vi "make_scene_main.vi"(1 "All Properties":T9, 5 "Scene Objects In":T2, 7 "Graph Properties":T1, 9 "Plot Processed Data":T3={"Plot Rep Arrays"=[], "Graph Range Min/Max"={"X"={"Min"=0.0, "Max"=-inf}, "Y"={"Min"=0.0, "Max"=-inf}, "Z"={"Min"=inf, "Max"=-inf}, "Amplitude"={"Min"=0.0, "Max"=0.0}}}, 12 "Update?":T35, 14 "Track Eye":T34) -> (6 "Scene Objects Out":T2, 10 "Translate By":T33, 15 "Scale By":T33)   [LabVIEW 2020, in "3DPC_SurfacePlot.xctl"]
uses:
  <vilib>/Native 3D Graph/xcontrol/3DPC_SurfacePlot.xctl
  <vilib>/Native 3D Graph/typedefs/vector.ctl
  <vilib>/Native 3D Graph/typedefs/update_scene_all.ctl
  <vilib>/Native 3D Graph/typedefs/update_scene_component.ctl
  <vilib>/Native 3D Graph/typedefs/track_eye.ctl
  <vilib>/Native 3D Graph/typedefs/all_non_graph_prop.ctl
  <vilib>/Native 3D Graph/typedefs/prop_plot_all_array.ctl
  <vilib>/Native 3D Graph/typedefs/prop_plot_all.ctl
  <vilib>/Native 3D Graph/typedefs/prop_plot_projection.ctl
  <vilib>/Native 3D Graph/typedefs/prop_plot_surface.ctl
  <vilib>/Native 3D Graph/typedefs/prop_plot_contour.ctl
  <vilib>/Native 3D Graph/typedefs/prop_plot_normal.ctl
  <vilib>/Native 3D Graph/typedefs/prop_plot_point_line.ctl
  <vilib>/Native 3D Graph/typedefs/prop_value_pair_all.ctl
  <vilib>/Native 3D Graph/typedefs/prop_value_pair_1d.ctl
  <vilib>/Native 3D Graph/typedefs/prop_axes_all.ctl
  <vilib>/Native 3D Graph/typedefs/prop_axes_grid.ctl
  <vilib>/Native 3D Graph/typedefs/prop_axes_ticks.ctl
  <vilib>/Native 3D Graph/typedefs/range_cluster.ctl
  <vilib>/Native 3D Graph/typedefs/min_max.ctl
  <vilib>/Native 3D Graph/typedefs/prop_axes_captions.ctl
  <vilib>/Native 3D Graph/typedefs/prop_axes_labels.ctl
  <vilib>/Native 3D Graph/typedefs/prop_axes_autorange.ctl
  <vilib>/Native 3D Graph/typedefs/prop_cursor_all_array.ctl
  <vilib>/Native 3D Graph/typedefs/prop_cursor_point.ctl
  <vilib>/Native 3D Graph/typedefs/prop_cursor_position.ctl
  <vilib>/Native 3D Graph/typedefs/prop_cursor_line.ctl
  <vilib>/Native 3D Graph/typedefs/prop_cursor_plane.ctl
  <vilib>/Native 3D Graph/typedefs/prop_cursor_text.ctl
  <vilib>/Native 3D Graph/typedefs/prop_format.ctl
  <vilib>/Native 3D Graph/typedefs/prop_lighting.ctl
  <vilib>/Native 3D Graph/typedefs/plot_processed_data.ctl
  <vilib>/Native 3D Graph/typedefs/plot_rep_array.ctl
  <vilib>/Native 3D Graph/typedefs/plot_rep.ctl
  <vilib>/Native 3D Graph/typedefs/plot_rep_mesh_data.ctl
  <vilib>/Native 3D Graph/typedefs/state_scene_objects.ctl
  <vilib>/Native 3D Graph/typedefs/prop_graph.ctl
  <vilib>/picture/3D Picture Control/Object/Create Object (name).vi
  <vilib>/picture/3D Picture Control/NI_3D Picture Control.lvlib
panel:
  out "Scene Objects Out":T2
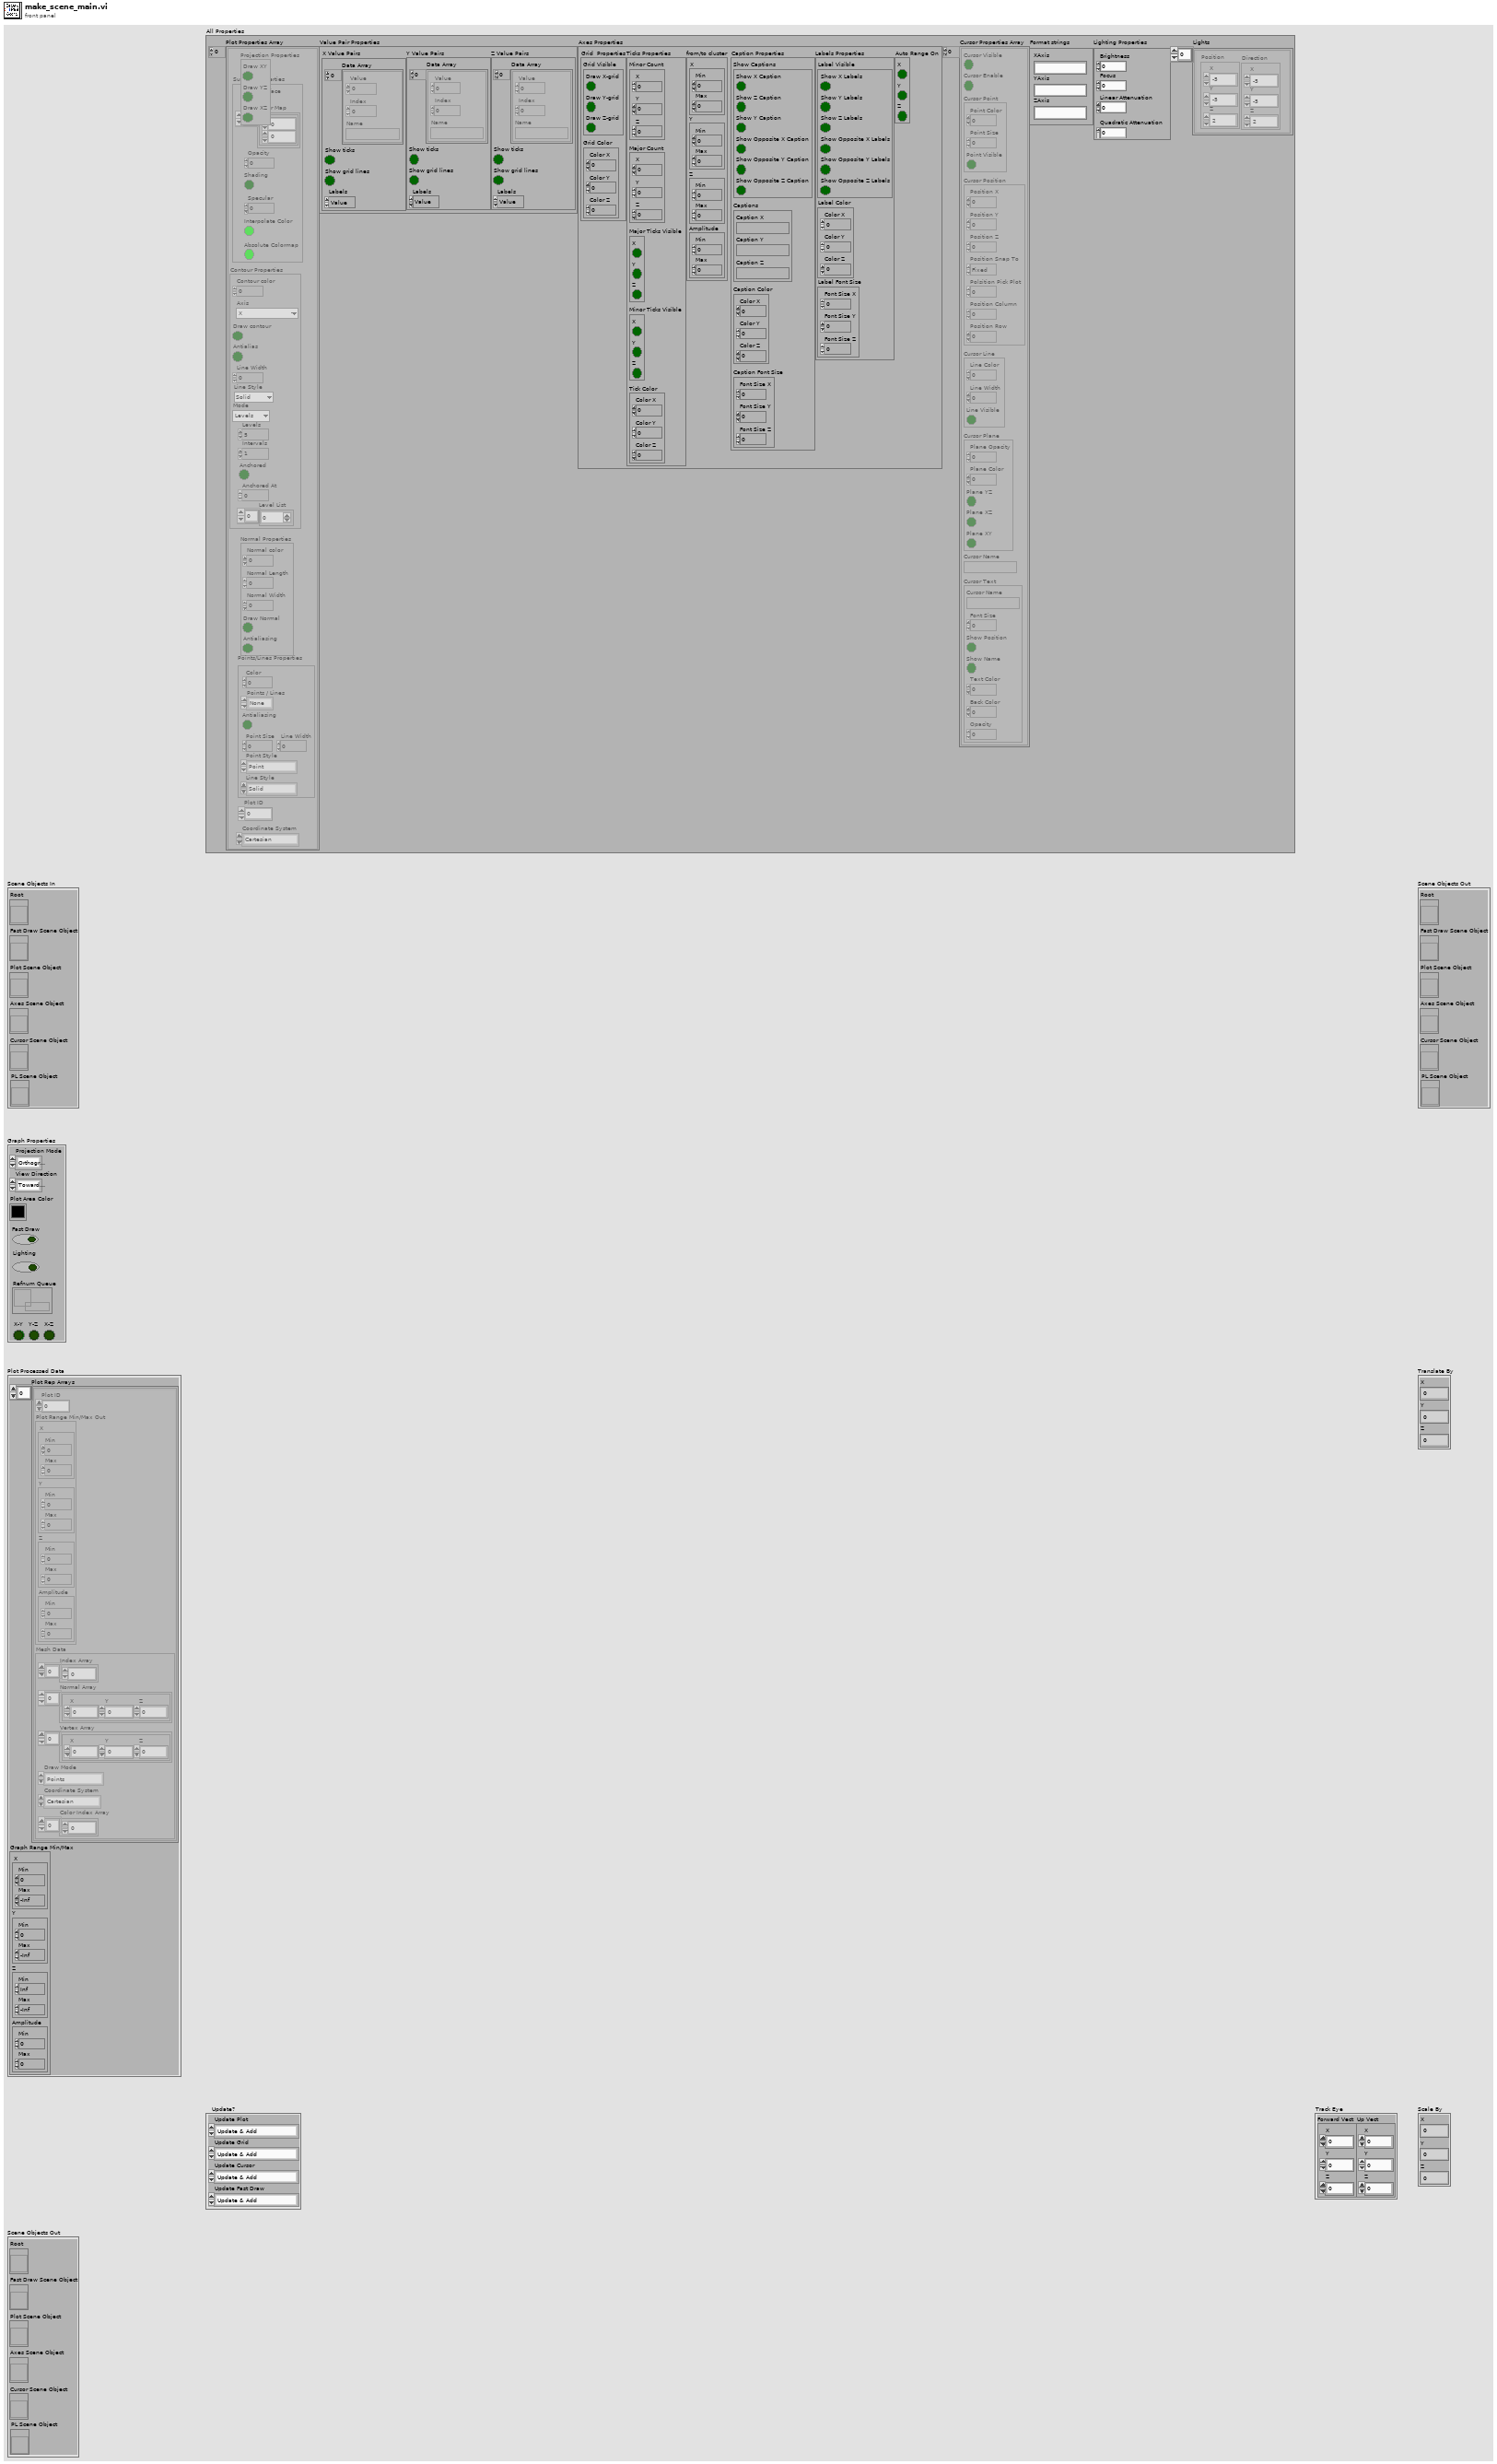
[diagram p1: front panel]
types:
  T1 = typedef "3DPC_SurfacePlot.xctl/prop_graph.ctl" = cluster{"Projection Mode":enum16{"Orthographic", "Perspective"}, "View Direction":enum32{"Towards X-Y Plane", "Towards Y-Z Plane", "Towards X-Z Plane", "User Define"}, "Plot Area Color":u32, "Fast Draw":bool, "X-Y":bool, "Y-Z":bool, "X-Z":bool, "Lighting":bool, "Refnum Queue":refnum<queue>}
  T2 = typedef "3DPC_SurfacePlot.xctl/state_scene_objects.ctl" = cluster{"Root":refnum<vi>, "Fast Draw Scene Object":refnum<vi>, "Plot Scene Object":refnum<vi>, "Axes Scene Object":refnum<vi>, "Cursor Scene Object":refnum<vi>, "PL Scene Object":refnum<vi>}
  T3 = typedef "plot_processed_data.ctl" = cluster{"Plot Rep Arrays":T4, "Graph Range Min/Max":T6}
  T4 = typedef "3DPC_SurfacePlot.xctl/plot_rep_array.ctl" = T5[]
  T5 = typedef "3DPC_SurfacePlot.xctl/plot_rep.ctl" = cluster{"Plot ID":i32, "Plot Range Min/Max Out":T6, "Mesh Data":T8}
  T6 = typedef "3DPC_SurfacePlot.xctl/range_cluster.ctl" = cluster{"X":T7, "Y":T7, "Z":T7, "Amplitude":T7}
  T7 = typedef "3DPC_SurfacePlot.xctl/min_max.ctl" = cluster{"Min":sgl, "Max":sgl}
  T8 = typedef "3DPC_SurfacePlot.xctl/plot_rep_mesh_data.ctl" = cluster{"Index Array":u32[], "Normal Array":cluster{"X":sgl, "Y":sgl, "Z":sgl}[], "Vertex Array":cluster{"X":sgl, "Y":sgl, "Z":sgl}[], "Draw Mode":enum16{"Points", "Lines", "Line Strip", "Line Loop", "Triangles", "Triangle Strip", "Triangle Fan", "Quads", "Quad Strip", "Polygon"}, "Coordinate System":enum16{"Cartesian", "Cylindrical", "Spherical"}, "Color Index Array":i32[]}
  T9 = typedef "3DPC_SurfacePlot.xctl/all_non_graph_prop.ctl" = cluster{"Plot Properties Array":T10, "Value Pair Properties":T17, "Axes Properties":T19, "Cursor Properties Array":T25, "Format strings":T31, "Lighting Properties":T32, "Lights":cluster{"Position":cluster{"X":sgl, "Y":sgl, "Z":sgl}, "Direction":cluster{"X":sgl, "Y":sgl, "Z":sgl}}[]}
  T10 = typedef "3DPC_SurfacePlot.xctl/prop_plot_all_array.ctl" = T11[]
  T11 = typedef "3DPC_SurfacePlot.xctl/prop_plot_all.ctl" = cluster{"Projection Properties":T12, "Surface Properties":T13, "Contour Properties":T14, "Normal Properties":T15, "Points/Lines Properties":T16, "Plot ID":i32, "Coordinate System":enum16{"Cartesian", "Cylindrical", "Spherical"}}
  T12 = typedef "3DPC_SurfacePlot.xctl/prop_plot_projection.ctl" = cluster{"Draw XY":bool, "Draw YZ":bool, "Draw XZ":bool}
  T13 = typedef "3DPC_SurfacePlot.xctl/prop_plot_surface.ctl" = cluster{"Draw surface":bool, "Opacity":dbl, "Shading":bool, "Specular":i32, "Color Map":cluster{dbl, u32}[], "Interpolate Color":bool, "Absolute Colormap":bool}
  T14 = typedef "3DPC_SurfacePlot.xctl/prop_plot_contour.ctl" = cluster{"Contour color":u32, "Axis":enum16{"X", "Y", "Z"}, "Draw contour":bool, "Antialias":bool, "Line Width":sgl, "Contour Line Style":enum16{"Solid", "Dash", "Dot", "Dash Dot"}, "Mode":enum16{"Levels", "Intervals", "Level List"}, "Levels":sgl, "Intervals":sgl, "Anchored At":sgl, "Anchored":bool, "Level List":dbl[]}
  T15 = typedef "3DPC_SurfacePlot.xctl/prop_plot_normal.ctl" = cluster{"Normal color":u32, "Normal Length":sgl, "Normal Width":sgl, "Draw Normal":bool, "Antialiasing":bool}
  T16 = typedef "3DPC_SurfacePlot.xctl/prop_plot_point_line.ctl" = cluster{"Color":u32, "Antialiasing":bool, "Point Size":sgl, "Points / Lines":enum16{"None", "Points", "Lines", "Both"}, "Point Style":enum16{"Point", "EmptySquare", "Asterisk", "Diamond", "EmptyCircle", "Circle", "X"}, "Line Style":enum16{"Solid", "Dash", "Dot", "Dash Dot"}, "Line Width":sgl}
  T17 = typedef "3DPC_SurfacePlot.xctl/prop_value_pair_all.ctl" = cluster{"X Value Pairs":cluster{"Data Array":cluster{"Value":sgl, "Index":i32, "Name":string}[], "Show ticks":bool, "Show grid lines":bool, "Labels":enum16{"Value", "None", "Name"}}, "Y Value Pairs":T18, "Z Value Pairs":T18}
  T18 = typedef "3DPC_SurfacePlot.xctl/prop_value_pair_1d.ctl" = cluster{"Data Array":cluster{"Value":sgl, "Index":i32, "Name":string}[], "Show ticks":bool, "Show grid lines":bool, "Labels":enum16{"Value", "None", "Name"}}
  T19 = typedef "3DPC_SurfacePlot.xctl/prop_axes_all.ctl" = cluster{"Grid  Properties":T20, "Ticks Properties":T21, "from/to cluster":T6, "Caption Properties":T22, "Labels Properties":T23, "Auto Range On":T24}
  T20 = typedef "3DPC_SurfacePlot.xctl/prop_axes_grid.ctl" = cluster{"Grid Visible":cluster{"Draw X-grid":bool, "Draw Y-grid":bool, "Draw Z-grid":bool}, "Grid Color":cluster{"Color X":u32, "Color Y":u32, "Color Z":u32}}
  T21 = typedef "3DPC_SurfacePlot.xctl/prop_axes_ticks.ctl" = cluster{"Minor Count":cluster{"X":i32, "Y":i32, "Z":i32}, "Major Count":cluster{"X":i32, "Y":i32, "Z":i32}, "Major Ticks Visible":cluster{"X":bool, "Y":bool, "Z":bool}, "Minor Ticks Visible":cluster{"X":bool, "Y":bool, "Z":bool}, "Tick Color":cluster{"Color X":u32, "Color Y":u32, "Color Z":u32}}
  T22 = typedef "3DPC_SurfacePlot.xctl/prop_axes_captions.ctl" = cluster{"Show Captions":cluster{"Show X Caption":bool, "Show Z Caption":bool, "Show Y Caption":bool, "Show Opposite X Caption":bool, "Show Opposite Y Caption":bool, "Show Opposite Z Caption":bool}, "Captions":cluster{"Caption X":string, "Caption Y":string, "Caption Z":string}, "Caption Color":cluster{"Color X":u32, "Color Y":u32, "Color Z":u32}, "Caption Font Size":cluster{"Font Size X":i16, "Font Size Y":i16, "Font Size Z":i16}}
  T23 = typedef "3DPC_SurfacePlot.xctl/prop_axes_labels.ctl" = cluster{"Label Visible":cluster{"Show X Labels":bool, "Show Y Labels":bool, "Show Z Labels":bool, "Show Opposite X Labels":bool, "Show Opposite Y Labels":bool, "Show Opposite Z Labels":bool}, "Label Color":cluster{"Color X":u32, "Color Y":u32, "Color Z":u32}, "Label Font Size":cluster{"Font Size X":i16, "Font Size Y":i16, "Font Size Z":i16}}
  T24 = typedef "3DPC_SurfacePlot.xctl/prop_axes_autorange.ctl" = cluster{"X":bool, "Y":bool, "Z":bool}
  T25 = typedef "3DPC_SurfacePlot.xctl/prop_cursor_all_array.ctl" = cluster{"Cursor Visible":bool, "Cursor Enable":bool, "Cursor Point":T26, "Cursor Position":T27, "Cursor Line":T28, "Cursor Plane":T29, "Cursor Name":string, "Cursor Text":T30}[]
  T26 = typedef "3DPC_SurfacePlot.xctl/prop_cursor_point.ctl" = cluster{"Point Color":u32, "Point Size":dbl, "Point Visible":bool}
  T27 = typedef "3DPC_SurfacePlot.xctl/prop_cursor_position.ctl" = cluster{"Position X":dbl, "Position Y":dbl, "Position Z":dbl, "Position Snap To":enum16{"Fixed", "Nearest Plot", "Snap to Plot"}, "Polsition Pick Plot":u16, "Position Column":i32, "Position Row":i32}
  T28 = typedef "3DPC_SurfacePlot.xctl/prop_cursor_line.ctl" = cluster{"Line Color":u32, "Line Width":dbl, "Line Visible":bool}
  T29 = typedef "3DPC_SurfacePlot.xctl/prop_cursor_plane.ctl" = cluster{"Plane Opacity":dbl, "Plane Color":u32, "Plane YZ":bool, "Plane XZ":bool, "Plane XY":bool}
  T30 = typedef "3DPC_SurfacePlot.xctl/prop_cursor_text.ctl" = cluster{"Cursor Name":string, "Font Size":i32, "Show Position":bool, "Show Name":bool, "Text Color":u32, "Back Color":u32, "Opacity":dbl}
  T31 = typedef "3DPC_SurfacePlot.xctl/prop_format.ctl" = cluster{"XAxis":string, "YAxis":string, "ZAxis":string}
  T32 = typedef "3DPC_SurfacePlot.xctl/prop_lighting.ctl" = cluster{"Brightness":i32, "Focus":dbl, "Linear Attenuation":dbl, "Quadratic Attenuation":dbl}
  T33 = typedef "3DPC_SurfacePlot.xctl/vector.ctl" = cluster{"X":sgl, "Y":sgl, "Z":sgl}
  T34 = typedef "3DPC_SurfacePlot.xctl/track_eye.ctl" = cluster{"Forward Vect":T33, "Up Vect":T33}
  T35 = typedef "3DPC_SurfacePlot.xctl/update_scene_all.ctl" = cluster{"Update Plot":T36, "Update Grid":T36, "Update Cursor":T36, "Update Fast Draw":T36}
  T36 = typedef "3DPC_SurfacePlot.xctl/update_scene_component.ctl" = enum16{"Update & Add", "Update & Not Add", "Remove ", "Nothing", "Add"}
  T37 = cluster{"Position":cluster{"X":sgl, "Y":sgl, "Z":sgl}, "Direction":cluster{"X":sgl, "Y":sgl, "Z":sgl}}[]
  T38 = enum16{"Points", "Lines", "Line Strip", "Line Loop", "Triangles", "Triangle Strip", "Triangle Fan", "Quads", "Quad Strip", "Polygon"}
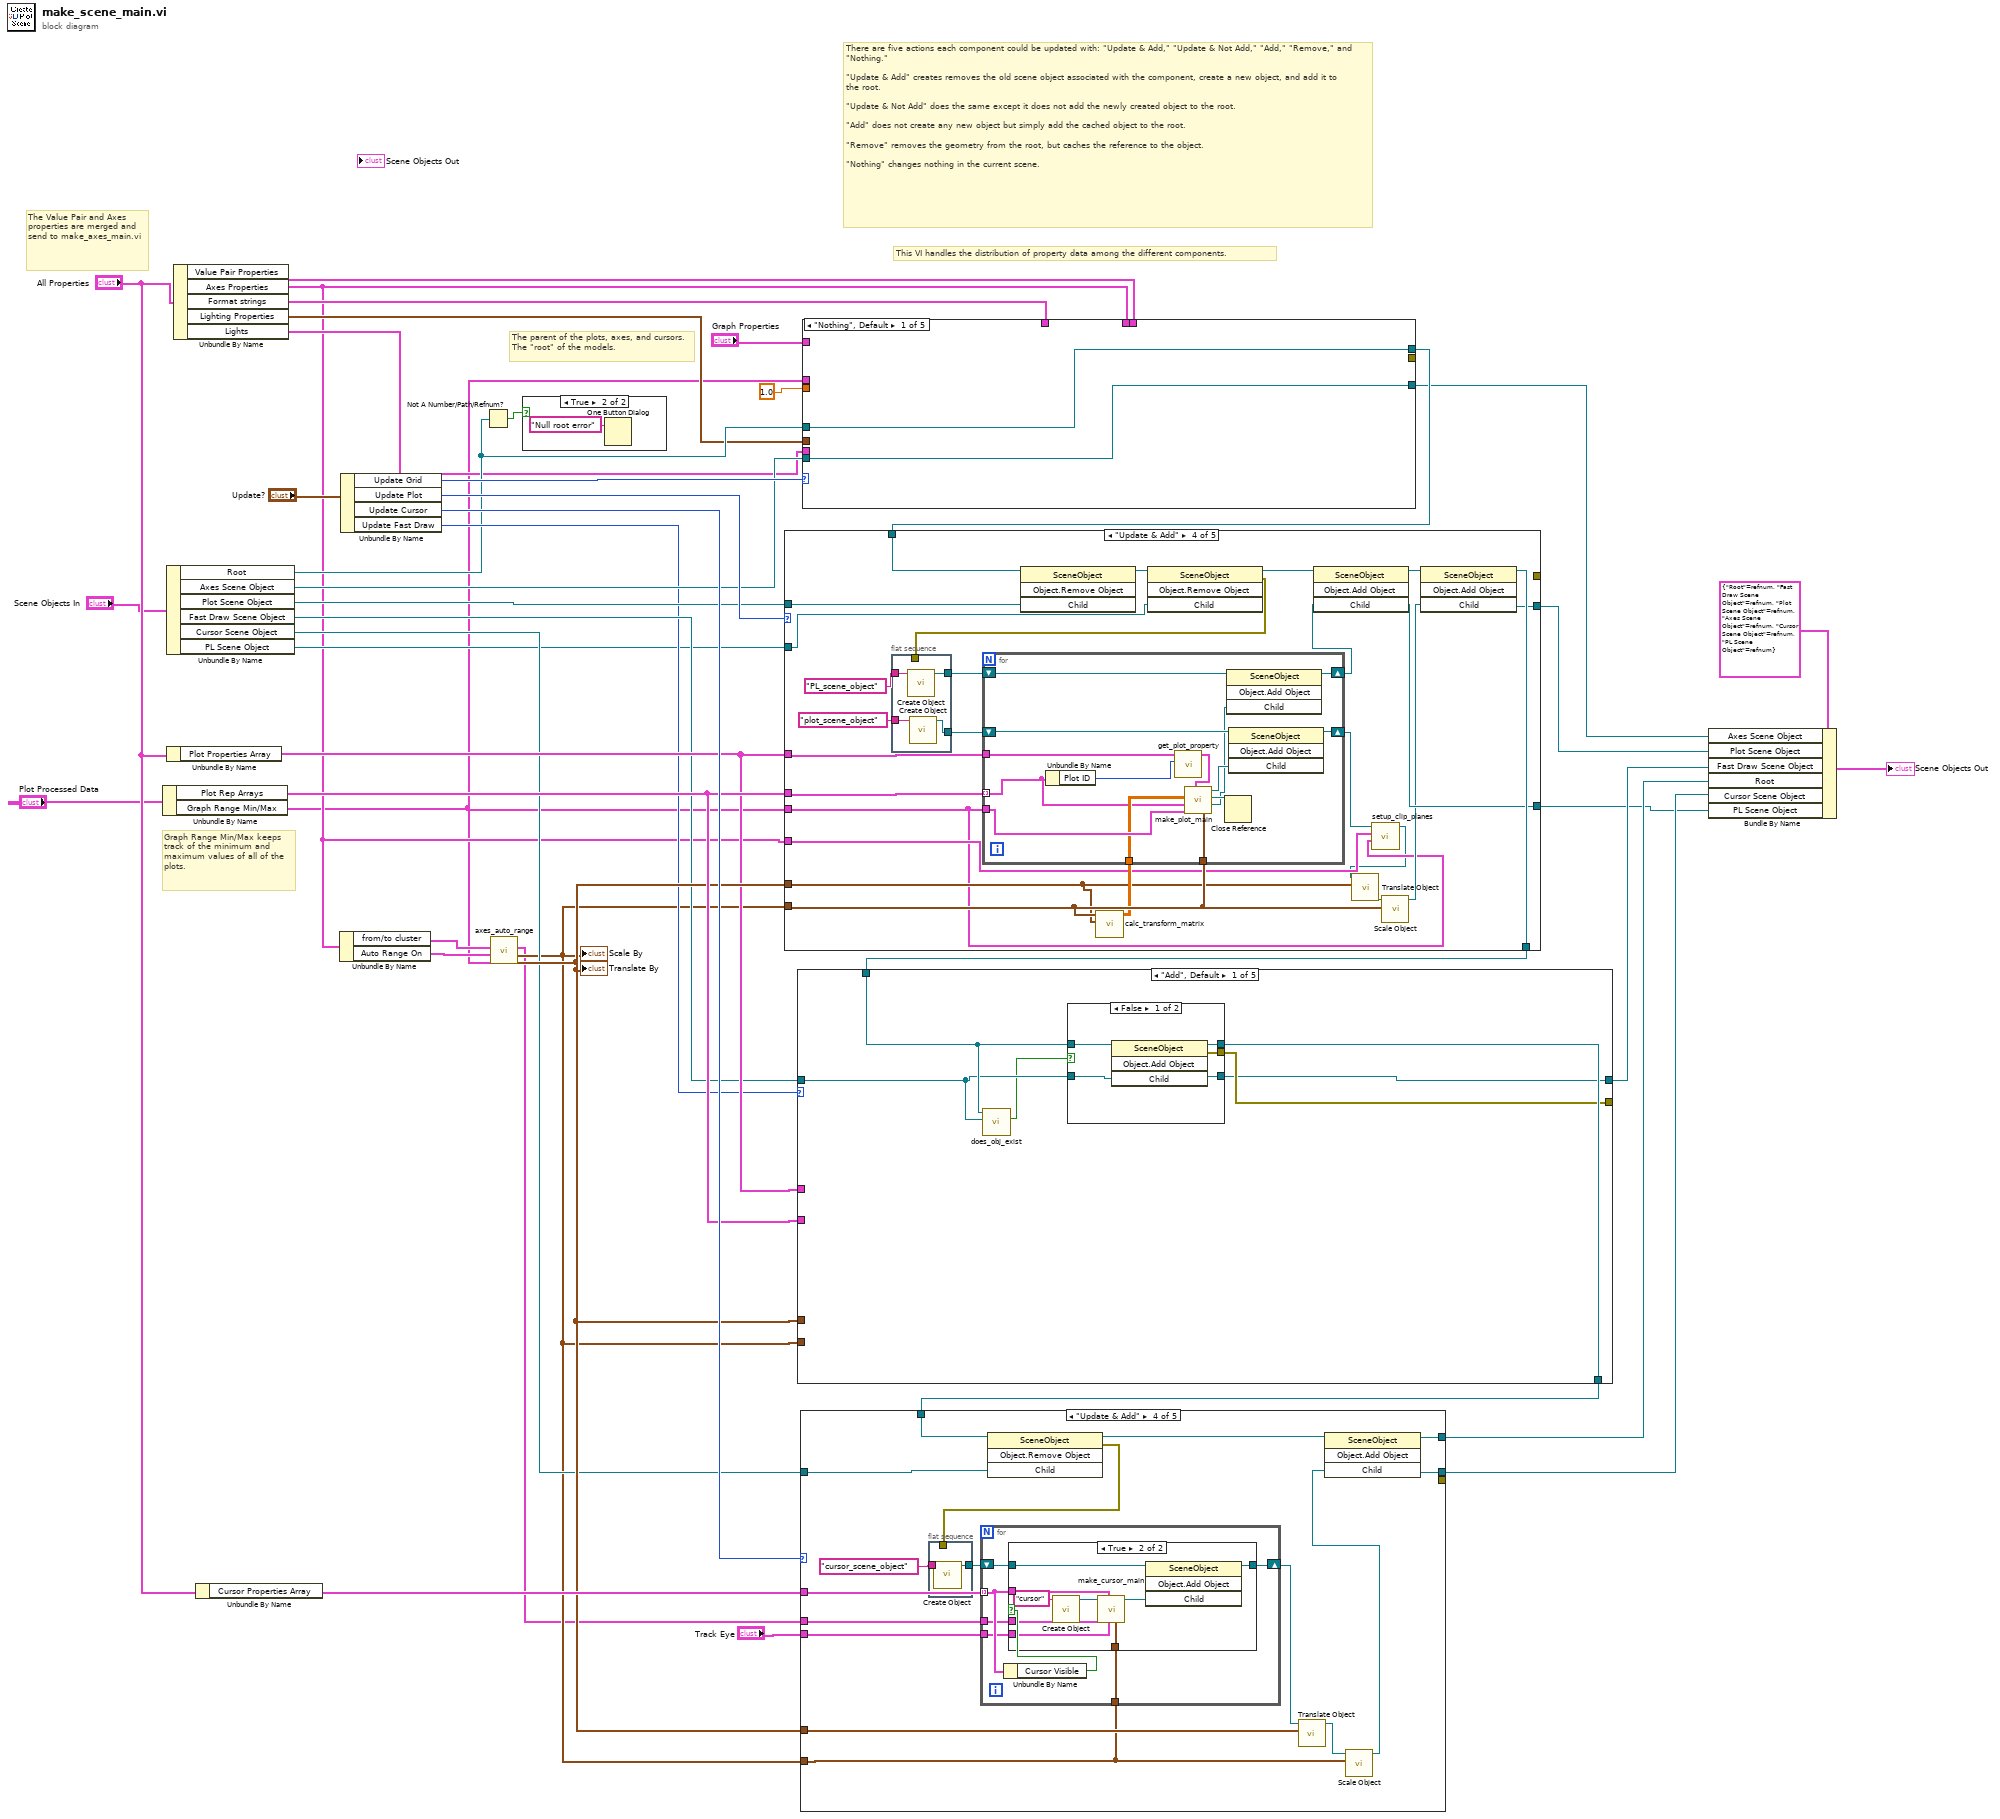
[diagram p0: block diagram]
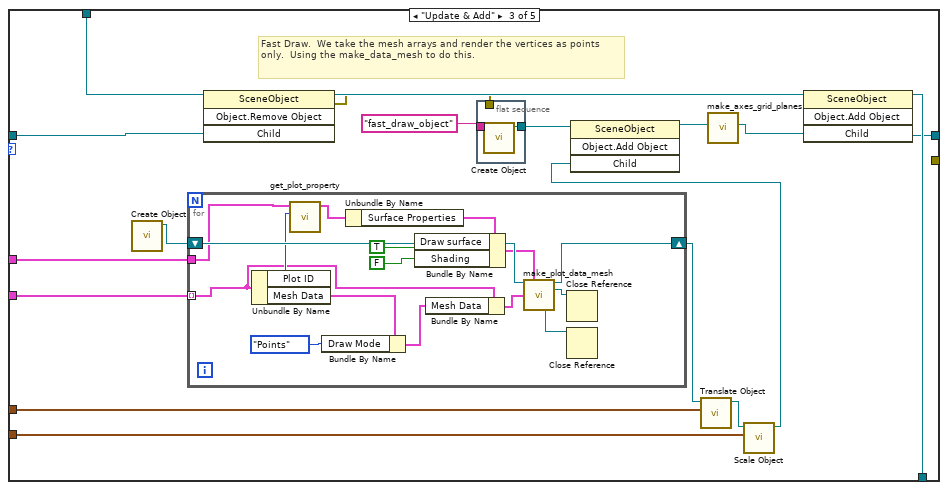
[diagram p5: hidden frame]
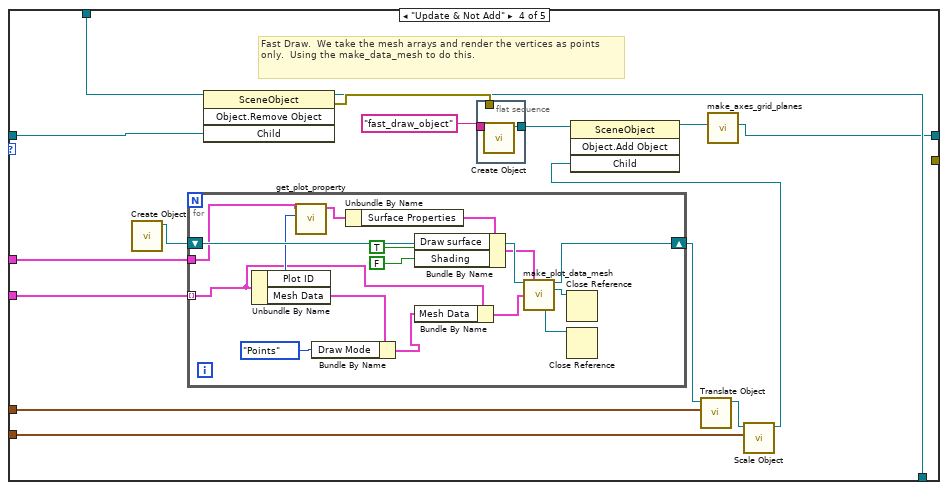
[diagram p6: hidden frame]
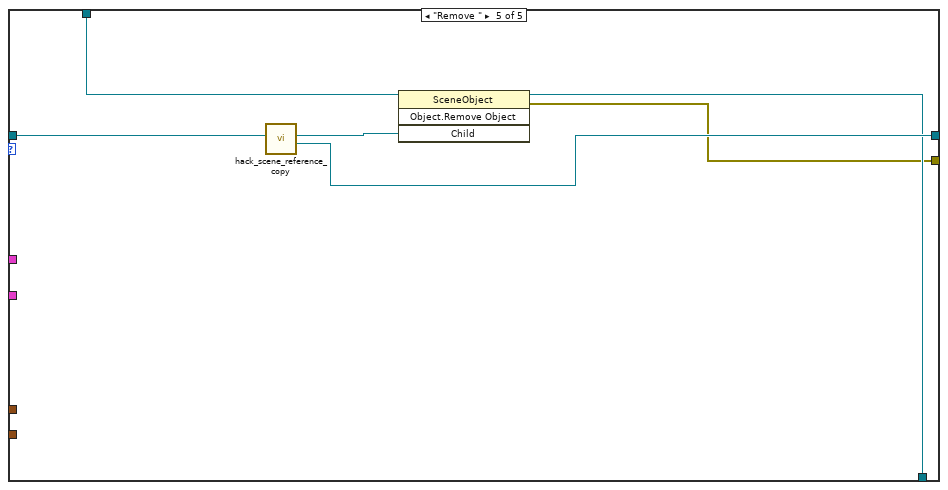
[diagram p7: hidden frame]
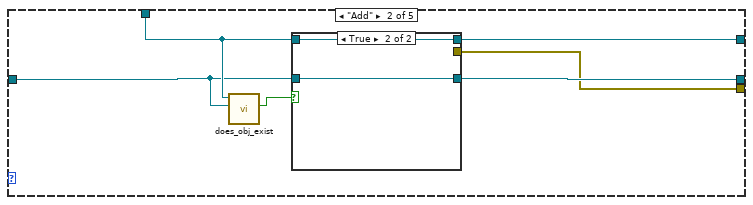
[diagram p9: hidden frame]
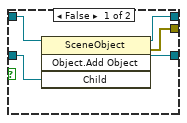
[diagram p10: hidden frame]
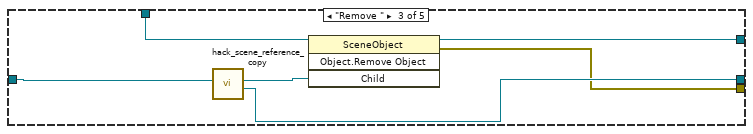
[diagram p11: hidden frame]
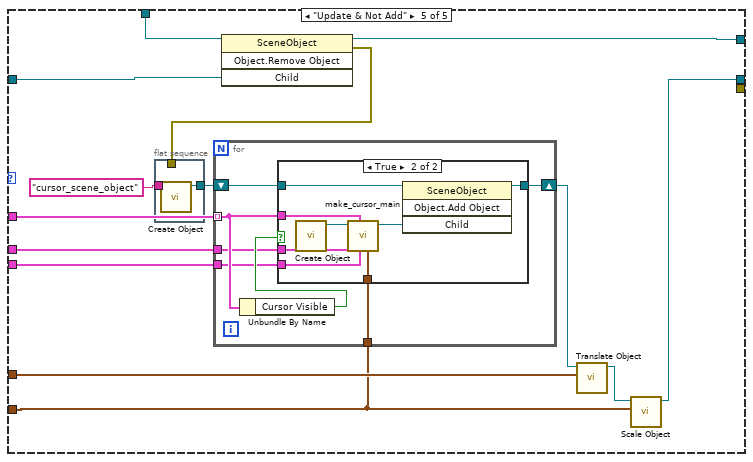
[diagram p13: hidden frame]
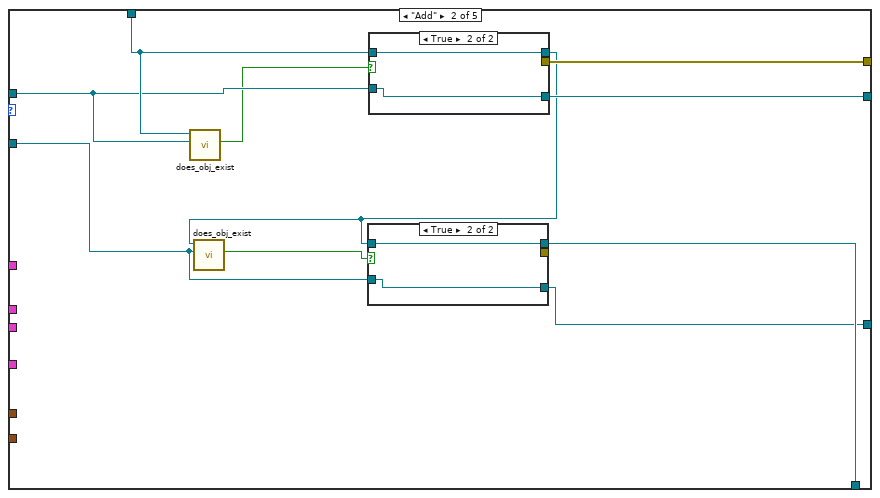
[diagram p16: hidden frame]
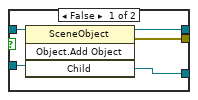
[diagram p17: hidden frame]
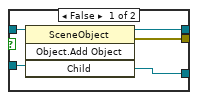
[diagram p18: hidden frame]
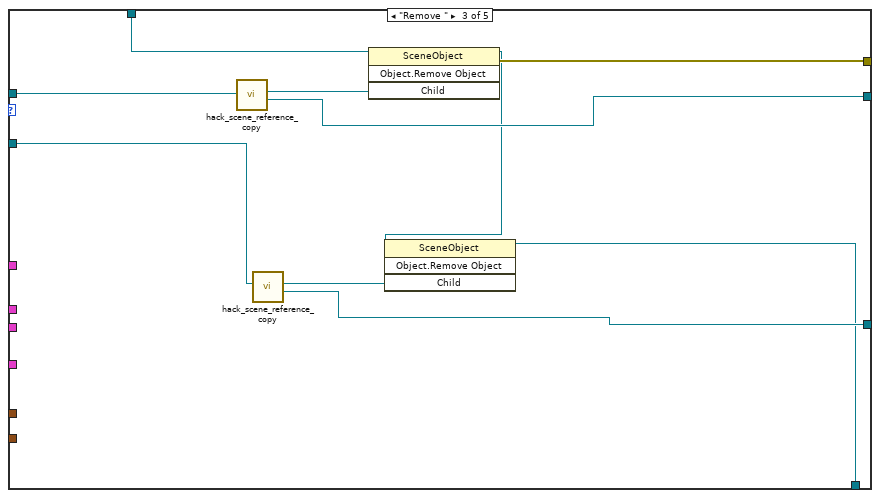
[diagram p19: hidden frame]
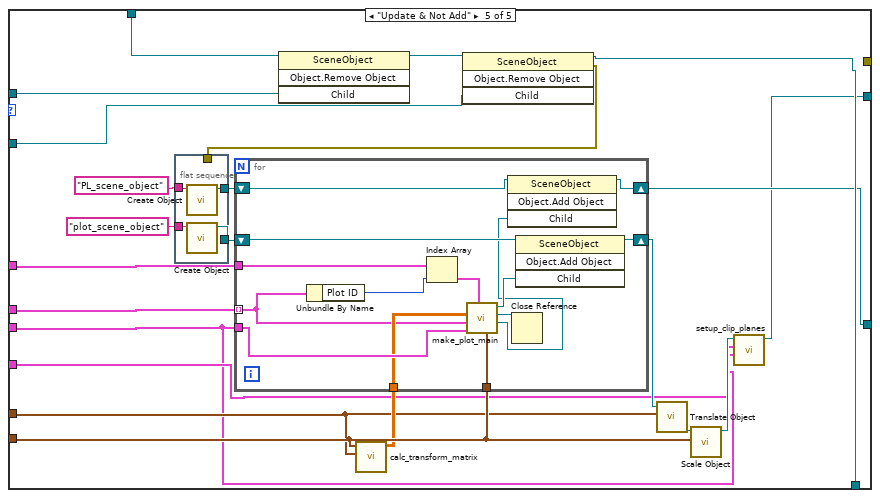
[diagram p20: hidden frame]
diagram:
  # "The parent of the plots, axes, and cursors.  The \"root\" of the models."
  # "There are five actions each component could be updated with: \"Update & Add,\" \"Update & Not Add,\" \"Add,\" \"Remove,\" and \"Nothing.\"  \n\n\"Update & Add\" creates removes the old scene object associated with the component, create a new object, and add it to the root.  \n\n\"Update & Not Add\" does the same except it does not add the newly created object to the root. \n\n\"Add\" does not create any new object but simply add the cached object to the root.   \n\n\"Remove\" removes the geometry from the root, but caches the reference to the object.\n\n\"Nothing\" changes nothing in the current scene."
  # "Graph Range Min/Max keeps track of the minimum and maximum values of all of the plots."
  # "The Value Pair and Axes properties are merged and send to make_axes_main.vi"
  # "This VI handles the distribution of property data among the different components."
  n1 = Unbundle By Name("Plot Processed Data") -> ("Plot Rep Arrays"=w29:T4, "Graph Range Min/Max"=w1:T6)
  n2 = Unbundle By Name("Scene Objects In") -> ("Root"=w13:refnum<vi>, "Axes Scene Object"=w19:refnum<vi>, "Plot Scene Object"=w18:refnum<vi>, "Fast Draw Scene Object"=w17:refnum<vi>, "Cursor Scene Object"=w16:refnum<vi>, "PL Scene Object"=w7:refnum<vi>)
  n3 = Unbundle By Name("All Properties") -> ("Plot Properties Array"=w27:T10)
  n4 = Unbundle By Name("All Properties") -> ("Value Pair Properties"=w35:T17, "Axes Properties"=w4:T19, "Format strings"=w11:T31, "Lighting Properties"=w10:T32, "Lights"=w9:T37)
  n5 = Unbundle By Name("All Properties") -> ("Cursor Properties Array"=w34:T25)
  n6 = Unbundle By Name(w4) -> ("from/to cluster"=w38:T6, "Auto Range On"=w37:T24)
  n7 = Unbundle By Name("Update?") -> ("Update Grid"=w42:T36, "Update Plot"=w41:T36, "Update Cursor"=w40:T36, "Update Fast Draw"=w15:T36)
  n8 = Not A Number/Path/Refnum?(number/path/refnum=w13) -> (NaN/Path/Refnum?=w12:bool)
  n9 = call <vilib>:"axes_auto_range.vi"("Acutal Range"=w1, "Auto Range On"=w37, "Set Range To"=w38) -> ("Translate"=w28:T33, "Scale"=w3:T33, "Range Min/Max"=w2:T6)  [unwired: 6 out]
  "Scale By" <- w3
  "Translate By" <- w28
  n10 = case shown="True" w12 {
    frame False {
    }
    frame True {
      n11 = One Button Dialog(message="Null root error") -> ()  [unwired: 2 out]
    }
  }
  n12 = case shown="\"Nothing\", Default" w42 {
    tunnel: 1.0 ("y") -> [_ _ _ w81 w99]
    tunnel: w35 -> [_ _ _ w80 w98]
    tunnel: w13 -> [w46 w52 w55 w66 w89]
    tunnel: [w46 w51 w57 w76 w90] -> w32
    tunnel: w4 -> [_ _ _ w75 w95]
    tunnel: w1 -> [_ _ _ w74 w94]
    tunnel: [w45 w48 w56 w71 w91] -> w22
    tunnel: w19 -> [w45 w50 w54 w69 w92]
    tunnel: [_ w47 _ _ _] -> _
    tunnel: w11 -> [_ _ _ w70 w84]
    tunnel: w10 -> [_ _ _ w68 w87]
    tunnel: w9 -> [_ _ _ w67 w86]
    tunnel: "Graph Properties" -> [_ _ _ w64 w85]
    frame "Nothing", Default {
    }
    frame "Remove " {
      n13 = call <vilib>:"hack_scene_reference_copy.vi"("Object   Orig In"=w50) -> ("Object Copy Out"=w48:refnum<vi>, "Object Orig Out"=w49:refnum<vi>)  [unwired: 9 out]
      n14 = invoke class="SceneObject" method="Object.Remove Object"(reference=w52, "Child"=w49) -> (reference out=w51:refnum<vi>, error out=w47:errorcluster)  [unwired: 2 in, 2 out]
    }
    frame "Add" {
      n15 = call <vilib>:"does_obj_exist.vi"("Plot Scene Object"=w54, "Root"=w55) -> ("obj exists"=w53:bool)  [unwired: 9 out]
      n16 = case shown="False" w53 {
        tunnel: [w61 w63] -> w57
        tunnel: [w60 w62] -> w56
        tunnel: w55 -> [w59 w63]
        tunnel: w54 -> [w58 w62]
        frame False {
          n17 = invoke class="SceneObject" method="Object.Add Object"(reference=w59, "Child"=w58) -> (reference out=w61:refnum<vi>, "Child"=w60:refnum<vi>)  [unwired: 2 in, 2 out]
        }
        frame True {
        }
      }
    }
    frame "Update & Add" {
      n18 = call <vilib>:"update_lights.vi"("Lights"=w67, "Lighting Properties"=w68, "Scene:New Object"=w66) -> ("Scene:New Object 2"=w65:refnum<vi>)  [unwired: 8 out]
      n19 = flat-sequence {
        tunnel: [w83] -> w79
        tunnel: "axes_scene_object" ("Name") -> [w82]
        tunnel: w72 -> [_]
        frame #0 {
          n20 = call-poly <vilib>:"Create Object.vi"("Name"=w82) -> ("Scene:New Object"=w83:refnum<vi>)  [unwired: 9 in, 1 out]
        }
      }
      n21 = invoke class="SceneObject" method="Object.Remove Object"(reference=w65, "Child"=w69) -> (reference out=w77:refnum<vi>, error out=w72:errorcluster)  [unwired: 2 in, 2 out]
      n22 = call <vilib>:"make_axes_main.vi"("Value Pair Properties"=w80, "Format strings"=w70, "Axes Properties"=w75, "length"=w81, "Range Min/Max"=w74, "Graph Properties"=w64, "Grid Scene Object In"=w79) -> ("Grid Scene Object Out"=w73:refnum<vi>)  [unwired: 4 out]
      n23 = invoke class="SceneObject" method="Object.Add Object"(reference=w77, "Child"=w73) -> (reference out=w76:refnum<vi>, "Child"=w71:refnum<vi>)  [unwired: 2 in, 2 out]
    }
    frame "Update & Not Add" {
      n24 = call <vilib>:"update_lights.vi"("Lights"=w86, "Lighting Properties"=w87, "Scene:New Object"=w89) -> ("Scene:New Object 2"=w88:refnum<vi>)  [unwired: 8 out]
      n25 = flat-sequence {
        tunnel: [w101] -> w97
        tunnel: "axes_scene_object" ("Name") -> [w100]
        tunnel: w93 -> [_]
        frame #0 {
          n26 = call-poly <vilib>:"Create Object.vi"("Name"=w100) -> ("Scene:New Object"=w101:refnum<vi>)  [unwired: 9 in, 1 out]
        }
      }
      n27 = invoke class="SceneObject" method="Object.Remove Object"(reference=w88, "Child"=w92) -> (reference out=w90:refnum<vi>, error out=w93:errorcluster)  [unwired: 2 in, 2 out]
      n28 = call <vilib>:"make_axes_main.vi"("Value Pair Properties"=w98, "Format strings"=w84, "Axes Properties"=w95, "length"=w99, "Range Min/Max"=w94, "Graph Properties"=w85, "Grid Scene Object In"=w97) -> ("Grid Scene Object Out"=w91:refnum<vi>)  [unwired: 4 out]
    }
  }
  n29 = case shown="\"Update & Add\"" w41 {
    tunnel: w32 -> [w104 w112 w138 w161 w199]
    tunnel: [w104 w109 w129 w164 w191] -> w31
    tunnel: w3 -> [_ _ _ w155 w194]
    tunnel: w28 -> [_ _ _ w144 w187]
    tunnel: w27 -> [_ _ _ w162 w201]
    tunnel: w29 -> [_ _ _ w156 w200]
    tunnel: w1 -> [_ _ _ w141 w183]
    tunnel: [w103 w114 w135 w160 w185] -> w23
    tunnel: w18 -> [w103 w111 w137 w159 w197]
    tunnel: [_ w113 w134 _ _] -> _
    tunnel: w7 -> [w102 w106 w132 w151 w190]
    tunnel: [w102 w105 w131 w145 w189] -> w6
    tunnel: w4 -> [_ _ _ w142 w184]
    frame "Nothing", Default {
    }
    frame "Add" {
      n30 = call <vilib>:"does_obj_exist.vi"("Plot Scene Object"=w111, "Root"=w112) -> ("obj exists"=w110:bool)  [unwired: 9 out]
      n31 = case shown="True" w110 {
        tunnel: [w126 w127] -> w114
        tunnel: [w125 w128] -> w107
        tunnel: [w124 _] -> w113
        tunnel: w112 -> [w123 w128]
        tunnel: w111 -> [w122 w127]
        frame False {
          n32 = invoke class="SceneObject" method="Object.Add Object"(reference=w123, "Child"=w122) -> (reference out=w125:refnum<vi>, error out=w124:errorcluster, "Child"=w126:refnum<vi>)  [unwired: 2 in, 1 out]
        }
        frame True {
        }
      }
      n33 = call <vilib>:"does_obj_exist.vi"("Plot Scene Object"=w106, "Root"=w107) -> ("obj exists"=w108:bool)  [unwired: 9 out]
      n34 = case shown="True" w108 {
        tunnel: [w119 w120] -> w105
        tunnel: [w118 w121] -> w109
        tunnel: [w117 _] -> _
        tunnel: w107 -> [w116 w121]
        tunnel: w106 -> [w115 w120]
        frame False {
          n35 = invoke class="SceneObject" method="Object.Add Object"(reference=w116, "Child"=w115) -> (reference out=w118:refnum<vi>, error out=w117:errorcluster, "Child"=w119:refnum<vi>)  [unwired: 2 in, 1 out]
        }
        frame True {
        }
      }
    }
    frame "Remove " {
      n36 = call <vilib>:"hack_scene_reference_copy.vi"("Object   Orig In"=w137) -> ("Object Copy Out"=w135:refnum<vi>, "Object Orig Out"=w136:refnum<vi>)  [unwired: 9 out]
      n37 = call <vilib>:"hack_scene_reference_copy.vi"("Object   Orig In"=w132) -> ("Object Copy Out"=w131:refnum<vi>, "Object Orig Out"=w133:refnum<vi>)  [unwired: 9 out]
      n38 = invoke class="SceneObject" method="Object.Remove Object"(reference=w138, "Child"=w136) -> (reference out=w130:refnum<vi>, error out=w134:errorcluster)  [unwired: 2 in, 2 out]
      n39 = invoke class="SceneObject" method="Object.Remove Object"(reference=w130, "Child"=w133) -> (reference out=w129:refnum<vi>)  [unwired: 2 in, 3 out]
    }
    frame "Update & Add" {
      n40 = flat-sequence {
        tunnel: "plot_scene_object" ("Name") -> [w168]
        tunnel: [w167] -> w158
        tunnel: "PL_scene_object" ("Name") -> [w166]
        tunnel: w150 -> [_]
        tunnel: [w165] -> w149
        frame #0 {
          n41 = call-poly <vilib>:"Create Object.vi"("Name"=w166) -> ("Scene:New Object"=w165:refnum<vi>)  [unwired: 9 in, 1 out]
          n42 = call-poly <vilib>:"Create Object.vi"("Name"=w168) -> ("Scene:New Object"=w167:refnum<vi>)  [unwired: 9 in, 1 out]
        }
      }
      n43 = invoke class="SceneObject" method="Object.Remove Object"(reference=w161, "Child"=w159) -> (reference out=w152:refnum<vi>)  [unwired: 2 in, 3 out]
      n44 = call <vilib>:"calc_transform_matrix.vi"("Translate"=w144, "Scale"=w155) -> ("Transformation"=w154:sgl[][])  [unwired: 9 out]
      n45 = for {
        tunnel: w162 -> [w176]
        tunnel: w156 -> [w169] mode=indexing
        shift-right: [w182] -> w140
        shift-left: w158 -> [w181]
        tunnel: w141 -> [w178]
        tunnel: w155 -> [w174]
        tunnel: w154 -> [w173]
        shift-right: [w170] -> w146
        shift-left: w149 -> [w172]
        n46 = Unbundle By Name(w169) -> ("Plot ID"=w175:i32)
        n47 = call <vilib>:"get_plot_property.vi"("Plot ID"=w175, "Plot Properties Array"=w176) -> ("element"=w177:T11)  [unwired: 1 in, 8 out]
        n48 = call <vilib>:"make_plot_main.vi"("Graph Scale By"=w174, "Plot Property"=w177, "Graph Range Min/Max"=w178, "Plot Representation"=w169, "PL Transformation"=w173) -> ("PL Scene Object Out"=w171:refnum<vi>, "Surface Mesh Out"=w179:refnum<vi>, "Plot Scene Object Out"=w180:refnum<vi>)  [unwired: 2 in, 2 out]
        n49 = Close Reference(reference=w179) -> ()  [unwired: 1 in, 1 out]
        n50 = invoke class="SceneObject" method="Object.Add Object"(reference=w172, "Child"=w171) -> (reference out=w170:refnum<vi>)  [unwired: 2 in, 3 out]
        n51 = invoke class="SceneObject" method="Object.Add Object"(reference=w181, "Child"=w180) -> (reference out=w182:refnum<vi>)  [unwired: 2 in, 3 out]
      }
      n52 = invoke class="SceneObject" method="Object.Remove Object"(reference=w152, "Child"=w151) -> (reference out=w148:refnum<vi>, error out=w150:errorcluster)  [unwired: 2 in, 2 out]
      n53 = invoke class="SceneObject" method="Object.Add Object"(reference=w148, "Child"=w146) -> (reference out=w147:refnum<vi>, "Child"=w145:refnum<vi>)  [unwired: 2 in, 2 out]
      n54 = call <vilib>:"setup_clip_planes.vi"("Graph Range Min/Max"=w141, "Axes Properties"=w142, "Scene.Object In"=w140) -> ("Scene.Object Out"=w139:refnum<vi>)  [unwired: 8 out]
      n55 = call <vilib>:"Translate Object.vi"("Translation"=w144, "Scene.Object In"=w139) -> ("Scene.Object Out"=w163:refnum<vi>)  [unwired: 1 in, 8 out]
      n56 = call <vilib>:"Scale Object.vi"("Scale"=w155, "Scene.Object In"=w163) -> ("Scene.Object Out"=w143:refnum<vi>)  [unwired: 1 in, 8 out]
      n57 = invoke class="SceneObject" method="Object.Add Object"(reference=w147, "Child"=w143) -> (reference out=w164:refnum<vi>, "Child"=w160:refnum<vi>)  [unwired: 2 in, 2 out]
    }
    frame "Update & Not Add" {
      n58 = flat-sequence {
        tunnel: "plot_scene_object" ("Name") -> [w208]
        tunnel: [w207] -> w202
        tunnel: "PL_scene_object" ("Name") -> [w206]
        tunnel: [w205] -> w195
        tunnel: w188 -> [_]
        frame #0 {
          n59 = call-poly <vilib>:"Create Object.vi"("Name"=w206) -> ("Scene:New Object"=w205:refnum<vi>)  [unwired: 9 in, 1 out]
          n60 = call-poly <vilib>:"Create Object.vi"("Name"=w208) -> ("Scene:New Object"=w207:refnum<vi>)  [unwired: 9 in, 1 out]
        }
      }
      n61 = invoke class="SceneObject" method="Object.Remove Object"(reference=w199, "Child"=w197) -> (reference out=w192:refnum<vi>)  [unwired: 2 in, 3 out]
      n62 = call <vilib>:"calc_transform_matrix.vi"("Translate"=w187, "Scale"=w194) -> ("Transformation"=w193:sgl[][])  [unwired: 9 out]
      n63 = for {
        tunnel: w201 -> [w219]
        tunnel: w200 -> [w209] mode=indexing
        shift-right: [w222] -> w204
        shift-left: w202 -> [w221]
        tunnel: w183 -> [w215]
        tunnel: w194 -> [w214]
        shift-right: [w212] -> w189
        shift-left: w195 -> [w213]
        tunnel: w193 -> [w210]
        n64 = Unbundle By Name(w209) -> ("Plot ID"=w218:i32)
        n65 = Index Array(array=w219, index=w218) -> (element=w217:T11)
        n66 = call <vilib>:"make_plot_main.vi"("Graph Scale By"=w214, "Plot Property"=w217, "Graph Range Min/Max"=w215, "Plot Representation"=w209, "PL Transformation"=w210) -> ("PL Scene Object Out"=w211:refnum<vi>, "Surface Mesh Out"=w216:refnum<vi>, "Plot Scene Object Out"=w220:refnum<vi>)  [unwired: 2 in, 2 out]
        n67 = invoke class="SceneObject" method="Object.Add Object"(reference=w213, "Child"=w211) -> (reference out=w212:refnum<vi>)  [unwired: 2 in, 3 out]
        n68 = Close Reference(reference=w216) -> ()  [unwired: 1 in, 1 out]
        n69 = invoke class="SceneObject" method="Object.Add Object"(reference=w221, "Child"=w220) -> (reference out=w222:refnum<vi>)  [unwired: 2 in, 3 out]
      }
      n70 = invoke class="SceneObject" method="Object.Remove Object"(reference=w192, "Child"=w190) -> (reference out=w191:refnum<vi>, error out=w188:errorcluster)  [unwired: 2 in, 2 out]
      n71 = call <vilib>:"Translate Object.vi"("Translation"=w187, "Scene.Object In"=w204) -> ("Scene.Object Out"=w203:refnum<vi>)  [unwired: 1 in, 8 out]
      n72 = call <vilib>:"Scale Object.vi"("Scale"=w194, "Scene.Object In"=w203) -> ("Scene.Object Out"=w186:refnum<vi>)  [unwired: 1 in, 8 out]
      n73 = call <vilib>:"setup_clip_planes.vi"("Graph Range Min/Max"=w183, "Axes Properties"=w184, "Scene.Object In"=w186) -> ("Scene.Object Out"=w185:refnum<vi>)  [unwired: 8 out]
    }
  }
  n74 = case shown="\"Add\", Default" w15 {
    tunnel: w31 -> [w225 w237 w248 w284 w312]
    tunnel: [w228 w237 w254 w275 w309] -> w30
    tunnel: w3 -> [_ _ w253 w288 _]
    tunnel: w28 -> [_ _ w252 w287 _]
    tunnel: [w227 _ _ _ w308] -> _
    tunnel: w29 -> [_ _ w247 w283 _]
    tunnel: w27 -> [_ _ w246 w282 _]
    tunnel: [w226 w236 w244 w274 w310] -> w24
    tunnel: w17 -> [w224 w236 w243 w280 w311]
    frame "Add", Default {
      n75 = call <vilib>:"does_obj_exist.vi"("Plot Scene Object"=w224, "Root"=w225) -> ("obj exists"=w223:bool)  [unwired: 9 out]
      n76 = case shown="False" w223 {
        tunnel: w225 -> [w233 w235]
        tunnel: [w232 w235] -> w228
        tunnel: [w231 _] -> w227
        tunnel: w224 -> [w230 w234]
        tunnel: [w229 w234] -> w226
        frame False {
          n77 = invoke class="SceneObject" method="Object.Add Object"(reference=w233, "Child"=w230) -> (reference out=w232:refnum<vi>, error out=w231:errorcluster, "Child"=w229:refnum<vi>)  [unwired: 2 in, 1 out]
        }
        frame True {
        }
      }
    }
    frame "Nothing" {
    }
    frame "Update & Add" {
      # "Fast Draw.  We take the mesh arrays and render the vertices as points only.  Using the make_data_mesh to do this."
      n78 = call-poly <vilib>:"Create Object.vi"() -> ("Scene:New Object"=w242:refnum<vi>)  [unwired: 10 in, 1 out]
      n79 = for {
        tunnel: w247 -> [w260] mode=indexing
        tunnel: w246 -> [w263]
        shift-right: [w272] -> w251
        shift-left: w242 -> [w273]
        n80 = Unbundle By Name(w260) -> ("Plot ID"=w262:i32, "Mesh Data"=w265:T8)
        n81 = call <vilib>:"get_plot_property.vi"("Plot ID"=w262, "Plot Properties Array"=w263) -> ("element"=w261:T11)  [unwired: 1 in, 8 out]
        n82 = Bundle By Name(cluster=w265, "Draw Mode"=T38."Points") -> (w259:T8)
        n83 = Unbundle By Name(w261) -> ("Surface Properties"=w271:T13)
        n84 = Bundle By Name(cluster=w271, "Draw surface"=TRUE, "Shading"=FALSE ("Draw surface")) -> (w268:T13)
        n85 = Bundle By Name(cluster=w260, "Mesh Data"=w259) -> (w258:T5)
        n86 = call <vilib>:"make_plot_data_mesh.vi"("Scene:In Object"=w273, "Surface Properties"=w268, "Plot Representation"=w258) -> ("Collection Scene Object"=w272:refnum<vi>, "Data Mesh Out"=w267:refnum<vi>, "Data Scene Object Out"=w266:refnum<vi>)  [unwired: 4 in, 6 out]
        n87 = Close Reference(reference=w267) -> ()  [unwired: 1 in, 1 out]
        n88 = Close Reference(reference=w266) -> ()  [unwired: 1 in, 1 out]
      }
      n89 = invoke class="SceneObject" method="Object.Remove Object"(reference=w248, "Child"=w243) -> (reference out=w249:refnum<vi>, error out=w245:errorcluster)  [unwired: 2 in, 2 out]
      n90 = flat-sequence {
        tunnel: "fast_draw_object" ("Name") -> [w257]
        tunnel: w245 -> [_]
        tunnel: [w256] -> w241
        frame #0 {
          n91 = call-poly <vilib>:"Create Object.vi"("Name"=w257) -> ("Scene:New Object"=w256:refnum<vi>)  [unwired: 9 in, 1 out]
        }
      }
      n92 = call <vilib>:"Translate Object.vi"("Translation"=w252, "Scene.Object In"=w251) -> ("Scene.Object Out"=w250:refnum<vi>)  [unwired: 1 in, 8 out]
      n93 = call <vilib>:"Scale Object.vi"("Scale"=w253, "Scene.Object In"=w250) -> ("Scene.Object Out"=w240:refnum<vi>)  [unwired: 1 in, 8 out]
      n94 = invoke class="SceneObject" method="Object.Add Object"(reference=w241, "Child"=w240) -> (reference out=w239:refnum<vi>)  [unwired: 2 in, 3 out]
      n95 = call <vilib>:"make_axes_grid_planes.vi"("Scene Object In"=w239) -> ("Scene Object Out"=w238:refnum<vi>)  [unwired: 10 out]
      n96 = invoke class="SceneObject" method="Object.Add Object"(reference=w249, "Child"=w238) -> (reference out=w254:refnum<vi>, "Child"=w244:refnum<vi>)  [unwired: 2 in, 2 out]
    }
    frame "Update & Not Add" {
      # "Fast Draw.  We take the mesh arrays and render the vertices as points only.  Using the make_data_mesh to do this."
      n97 = call-poly <vilib>:"Create Object.vi"() -> ("Scene:New Object"=w279:refnum<vi>)  [unwired: 10 in, 1 out]
      n98 = for {
        tunnel: w283 -> [w292] mode=indexing
        tunnel: w282 -> [w296]
        shift-right: [w306] -> w286
        shift-left: w279 -> [w307]
        n99 = Unbundle By Name(w292) -> ("Plot ID"=w297:i32, "Mesh Data"=w299:T8)
        n100 = call <vilib>:"get_plot_property.vi"("Plot ID"=w297, "Plot Properties Array"=w296) -> ("element"=w295:T11)  [unwired: 1 in, 8 out]
        n101 = Bundle By Name(cluster=w299, "Draw Mode"=T38."Points") -> (w294:T8)
        n102 = Unbundle By Name(w295) -> ("Surface Properties"=w305:T13)
        n103 = Bundle By Name(cluster=w305, "Draw surface"=TRUE, "Shading"=FALSE ("Draw surface")) -> (w302:T13)
        n104 = Bundle By Name(cluster=w292, "Mesh Data"=w294) -> (w293:T5)
        n105 = call <vilib>:"make_plot_data_mesh.vi"("Scene:In Object"=w307, "Surface Properties"=w302, "Plot Representation"=w293) -> ("Collection Scene Object"=w306:refnum<vi>, "Data Mesh Out"=w301:refnum<vi>, "Data Scene Object Out"=w300:refnum<vi>)  [unwired: 3 in, 7 out]
        n106 = Close Reference(reference=w301) -> ()  [unwired: 1 in, 1 out]
        n107 = Close Reference(reference=w300) -> ()  [unwired: 1 in, 1 out]
      }
      n108 = invoke class="SceneObject" method="Object.Remove Object"(reference=w284, "Child"=w280) -> (reference out=w275:refnum<vi>, error out=w281:errorcluster)  [unwired: 2 in, 2 out]
      n109 = flat-sequence {
        tunnel: "fast_draw_object" ("Name") -> [w291]
        tunnel: w281 -> [_]
        tunnel: [w290] -> w278
        frame #0 {
          n110 = call-poly <vilib>:"Create Object.vi"("Name"=w291) -> ("Scene:New Object"=w290:refnum<vi>)  [unwired: 9 in, 1 out]
        }
      }
      n111 = call <vilib>:"Translate Object.vi"("Translation"=w287, "Scene.Object In"=w286) -> ("Scene.Object Out"=w285:refnum<vi>)  [unwired: 1 in, 8 out]
      n112 = call <vilib>:"Scale Object.vi"("Scale"=w288, "Scene.Object In"=w285) -> ("Scene.Object Out"=w277:refnum<vi>)  [unwired: 1 in, 8 out]
      n113 = invoke class="SceneObject" method="Object.Add Object"(reference=w278, "Child"=w277) -> (reference out=w276:refnum<vi>)  [unwired: 2 in, 3 out]
      n114 = call <vilib>:"make_axes_grid_planes.vi"("Scene Object In"=w276) -> ("Scene Object Out"=w274:refnum<vi>)  [unwired: 10 out]
    }
    frame "Remove " {
      n115 = call <vilib>:"hack_scene_reference_copy.vi"("Object   Orig In"=w311) -> ("Object Copy Out"=w310:refnum<vi>, "Object Orig Out"=w313:refnum<vi>)  [unwired: 9 out]
      n116 = invoke class="SceneObject" method="Object.Remove Object"(reference=w312, "Child"=w313) -> (reference out=w309:refnum<vi>, error out=w308:errorcluster)  [unwired: 2 in, 2 out]
    }
  }
  n117 = case shown="\"Update & Add\"" w40 {
    tunnel: w30 -> [w315 w318 w333 w346 w381]
    tunnel: w34 -> [_ _ _ w349 w383]
    tunnel: [w315 w321 w331 w347 w371] -> w25
    tunnel: "Track Eye" -> [_ _ _ w345 w380]
    tunnel: w3 -> [_ _ _ w335 w376]
    tunnel: w28 -> [_ _ _ w344 w379]
    tunnel: w2 -> [_ _ _ w341 w375]
    tunnel: [w314 w320 w330 w337 w370] -> w21
    tunnel: w16 -> [w314 w317 w332 w336 w372]
    tunnel: [_ w319 w329 _ _] -> _
    frame "Nothing", Default {
    }
    frame "Add" {
      n118 = call <vilib>:"does_obj_exist.vi"("Plot Scene Object"=w317, "Root"=w318) -> ("obj exists"=w316:bool)  [unwired: 9 out]
      n119 = case shown="True" w316 {
        tunnel: [w326 w328] -> w321
        tunnel: [w325 w327] -> w320
        tunnel: [w324 _] -> w319
        tunnel: w318 -> [w323 w328]
        tunnel: w317 -> [w322 w327]
        frame False {
          n120 = invoke class="SceneObject" method="Object.Add Object"(reference=w323, "Child"=w322) -> (reference out=w326:refnum<vi>, error out=w324:errorcluster, "Child"=w325:refnum<vi>)  [unwired: 2 in, 1 out]
        }
        frame True {
        }
      }
    }
    frame "Remove " {
      n121 = call <vilib>:"hack_scene_reference_copy.vi"("Object   Orig In"=w332) -> ("Object Copy Out"=w330:refnum<vi>, "Object Orig Out"=w334:refnum<vi>)  [unwired: 9 out]
      n122 = invoke class="SceneObject" method="Object.Remove Object"(reference=w333, "Child"=w334) -> (reference out=w331:refnum<vi>, error out=w329:errorcluster)  [unwired: 2 in, 2 out]
    }
    frame "Update & Add" {
      n123 = flat-sequence {
        tunnel: [w352] -> w348
        tunnel: "cursor_scene_object" ("Name") -> [w351]
        tunnel: w338 -> [_]
        frame #0 {
          n124 = call-poly <vilib>:"Create Object.vi"("Name"=w351) -> ("Scene:New Object"=w352:refnum<vi>)  [unwired: 9 in, 1 out]
        }
      }
      n125 = for {
        tunnel: w349 -> [w357] mode=indexing
        shift-right: [w358] -> w343
        shift-left: w348 -> [w359]
        tunnel: w345 -> [w355]
        tunnel: w335 -> [w354]
        tunnel: w341 -> [w353]
        n126 = Unbundle By Name(w357) -> ("Cursor Visible"=w356:bool)
        n127 = case shown="True" w356 {
          tunnel: w359 -> [w360 w368]
          tunnel: [w360 w366] -> w358
          tunnel: w357 -> [_ w364]
          tunnel: w355 -> [_ w365]
          tunnel: w354 -> [_ w363]
          tunnel: w353 -> [_ w362]
          frame False {
          }
          frame True {
            n128 = call-poly <vilib>:"Create Object.vi"("Name"="cursor") -> ("Scene:New Object"=w369:refnum<vi>)  [unwired: 9 in, 1 out]
            n129 = call <vilib>:"make_cursor_main.vi"("Scale"=w363, "Track Eye"=w365, "Cursor Properties"=w364, "Actual Range Min/Max"=w362, "Scene Cursor Object In"=w369) -> ("Scene Cursor Object Out"=w367:refnum<vi>)  [unwired: 1 in, 5 out]
            n130 = invoke class="SceneObject" method="Object.Add Object"(reference=w368, "Child"=w367) -> (reference out=w366:refnum<vi>)  [unwired: 2 in, 3 out]
          }
        }
      }
      n131 = invoke class="SceneObject" method="Object.Remove Object"(reference=w346, "Child"=w336) -> (reference out=w350:refnum<vi>, error out=w338:errorcluster)  [unwired: 2 in, 2 out]
      n132 = call <vilib>:"Translate Object.vi"("Translation"=w344, "Scene.Object In"=w343) -> ("Scene.Object Out"=w342:refnum<vi>)  [unwired: 1 in, 8 out]
      n133 = call <vilib>:"Scale Object.vi"("Scale"=w335, "Scene.Object In"=w342) -> ("Scene.Object Out"=w340:refnum<vi>)  [unwired: 1 in, 8 out]
      n134 = invoke class="SceneObject" method="Object.Add Object"(reference=w350, "Child"=w340) -> (reference out=w347:refnum<vi>, "Child"=w337:refnum<vi>)  [unwired: 2 in, 2 out]
    }
    frame "Update & Not Add" {
      n135 = flat-sequence {
        tunnel: [w385] -> w382
        tunnel: "cursor_scene_object" ("Name") -> [w384]
        tunnel: w373 -> [_]
        frame #0 {
          n136 = call-poly <vilib>:"Create Object.vi"("Name"=w384) -> ("Scene:New Object"=w385:refnum<vi>)  [unwired: 9 in, 1 out]
        }
      }
      n137 = for {
        tunnel: w383 -> [w390] mode=indexing
        shift-right: [w391] -> w378
        shift-left: w382 -> [w392]
        tunnel: w380 -> [w388]
        tunnel: w376 -> [w387]
        tunnel: w375 -> [w386]
        n138 = Unbundle By Name(w390) -> ("Cursor Visible"=w389:bool)
        n139 = case shown="True" w389 {
          tunnel: w392 -> [w393 w400]
          tunnel: [w393 w398] -> w391
          tunnel: w390 -> [_ w396]
          tunnel: w388 -> [_ w397]
          tunnel: w387 -> [_ w395]
          tunnel: w386 -> [_ w394]
          frame False {
          }
          frame True {
            n140 = call-poly <vilib>:"Create Object.vi"() -> ("Scene:New Object"=w401:refnum<vi>)  [unwired: 10 in, 1 out]
            n141 = call <vilib>:"make_cursor_main.vi"("Scale"=w395, "Track Eye"=w397, "Cursor Properties"=w396, "Actual Range Min/Max"=w394, "Scene Cursor Object In"=w401) -> ("Scene Cursor Object Out"=w399:refnum<vi>)  [unwired: 1 in, 5 out]
            n142 = invoke class="SceneObject" method="Object.Add Object"(reference=w400, "Child"=w399) -> (reference out=w398:refnum<vi>)  [unwired: 2 in, 3 out]
          }
        }
      }
      n143 = invoke class="SceneObject" method="Object.Remove Object"(reference=w381, "Child"=w372) -> (reference out=w371:refnum<vi>, error out=w373:errorcluster)  [unwired: 2 in, 2 out]
      n144 = call <vilib>:"Translate Object.vi"("Translation"=w379, "Scene.Object In"=w378) -> ("Scene.Object Out"=w377:refnum<vi>)  [unwired: 1 in, 8 out]
      n145 = call <vilib>:"Scale Object.vi"("Scale"=w376, "Scene.Object In"=w377) -> ("Scene.Object Out"=w370:refnum<vi>)  [unwired: 1 in, 8 out]
    }
  }
  n146 = Bundle By Name(cluster=T2 {"Root"=refnum, "Fast Draw Scene Object"=refnum, "Plot Scene Object"=refnum, "Axes Scene Object"=refnum, "Cursor Scene Object"=refnum, "PL Scene Object"=refnum} ("Scene Objects Out"), "Axes Scene Object"=w22, "Plot Scene Object"=w23, "Fast Draw Scene Object"=w24, "Root"=w25, "Cursor Scene Object"=w21, "PL Scene Object"=w6) -> (→"Scene Objects Out":T2)
